vi "Setup Monthly Folders.vi"() -> ()   [LabVIEW 2024]
uses:
  TypeDefs/comic--cluster.ctl
  <vilib>/addons/_JKI.lib/Serialization/JSON/JKI JSON Serialization.lvlib
  <userlib>/_OpenG.lib/string/string.llb/openg_string.lvlib
panel:
  out "multiples":string[](array[string])
  out "status":string
  out "error out":errorcluster
  in  "comic repo":path=path "D:/Comics/Marvel"
  in  "error in":errorcluster
  in  "path":path=path "D:/data/comics"
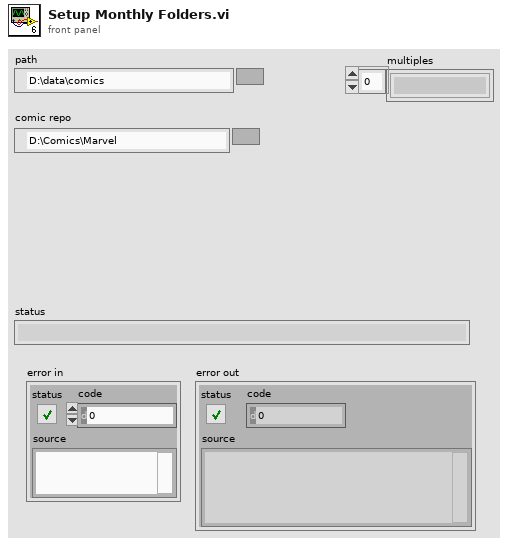
[diagram p1: front panel]
types:
  T1 = typedef "comic--cluster.ctl" = cluster{"id":i32, "digitalId":i32, "title":string, "issueNumber":i32, "variantDescription":string, "description":string, "modified":variant, "upc":string, "format":string, "pageCount":i32, "resourceURI":string, "urls":cluster{"type":string, "url":string}[], "series":cluster{"resourceURI":string, "name":string}, "dates":cluster{"type":string, "date":string}[], "prices":cluster{"price":dbl, "type":string}[], "thumbnail":cluster{"path":string, "extension":string}, "images":cluster{"path":string, "extension":string}[], "creators":cluster{"available":i32, "returned":i32, "collectionURI":string, "items":cluster{"resourceURI":string, "name":string, "role":string}[]}, "characters":cluster{"available":i32, "returned":i32, "collectionURI":string, "items":cluster{"resourceURI":string, "name":string}[]}, "stories":cluster{"available":i32, "returned":i32, "collectionURI":string, "items":cluster{"resourceURI":string, "name":string, "type":string}[]}, "events":cluster{"available":i32, "returned":i32, "collectionURI":string, "items":cluster{"resourceURI":string, "name":string}[]}}
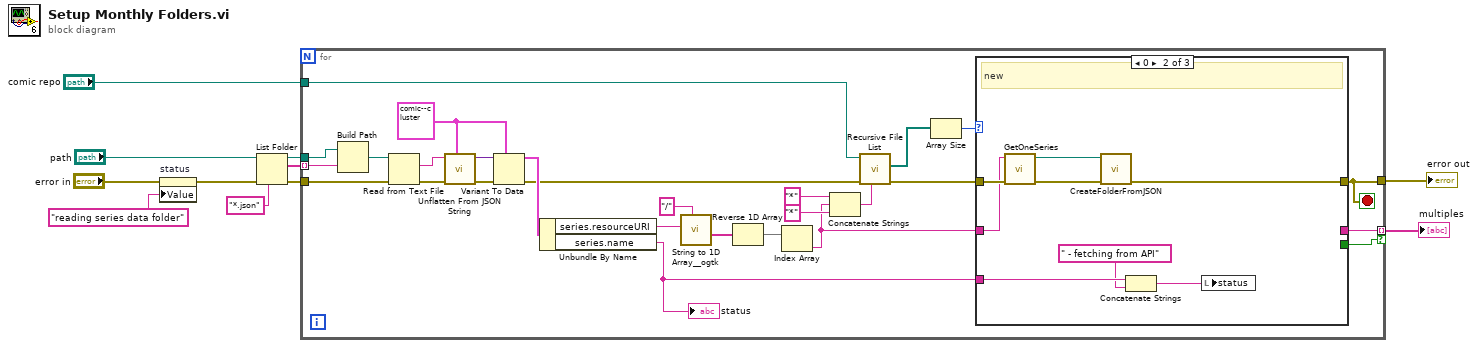
[diagram p0: block diagram]
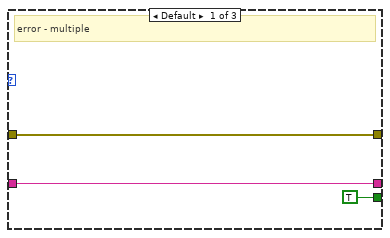
[diagram p2: hidden frame]
diagram:
  n1 = property on="status" class="Str"(error in="error in", "Value"="reading series data folder" ("status")) -> (error out=w2:errorcluster)  [unwired: 1 in, 1 out]
  n2 = List Folder(path="path", pattern="*.json", error in=w2) -> (path out=w7:path, filenames=w8:string[], error out=w9:errorcluster)  [unwired: 1 in, 1 out]
  n3 = for {
    tunnel: w9 -> [w36]
    tunnel: w8 -> [w38] mode=indexing
    tunnel: w7 -> [w37]
    tunnel: "comic repo" -> [w23]
    tunnel: [w16] -> w4
    tunnel: [w14] -> w5 mode=indexing if=w13
    stop <- w16 stop-if-true
    w30 = T1 {"id"=0, "digitalId"=0, "title"="", "issueNumber"=0, "variantDescription"="", "description"="", "modified"=variant, "upc"="", "format"="", "pageCount"=0, "resourceURI"="", "urls"=[], "series"={"resourceURI"="", "name"=""}, "dates"=[], "prices"=[], "thumbnail"={"path"="", "extension"=""}, "images"=[], "creators"={"available"=0, "returned"=0, "collectionURI"="", "items"=[]}, "characters"={"available"=0, "returned"=0, "collectionURI"="", "items"=[]}, "stories"={"available"=0, "returned"=0, "collectionURI"="", "items"=[]}, "events"={"available"=0, "returned"=0, "collectionURI"="", "items"=[]}} ("Cluster")
    n4 = Build Path(base path=w37, name or relative path=w38) -> (appended path=w35:path)
    n5 = Read from Text File(file (use dialog)=w35, error in=w36) -> (text=w33:string, error out=w34:errorcluster)  [unwired: 2 in, 2 out]
    n6 = call <vilib>:"Unflatten From JSON String.vi"("Type and Defaults"=w30, "error in (no error)"=w34, "JSON String"=w33) -> ("error out"=w32:errorcluster, "Variant"=w31:variant)  [unwired: 7 in]
    n7 = Variant To Data(error in=w32, type=w30, Variant=w31) -> (data=w29:T1, error out=w24:errorcluster)
    n8 = Unbundle By Name(w29) -> ("series.resourceURI"=w28:string, "series.name"=w12:string)
    "status" <- w12
    n9 = call <userlib>:"String to 1D Array__ogtk.vi"("delimiter (Tab)"="/", "string"=w28) -> ("Array of Strings"=w26:string[])  [unwired: 9 in]
    n10 = Reverse 1D Array(array=w26) -> (reversed array=w25:string[])
    n11 = Index Array(array=w25) -> (element=w15:string)  [unwired: 1 in]
    n12 = Concatenate Strings("*" ("string"), w15, "*" ("string")) -> (w22:string)
    n13 = call <vilib>:"Recursive File List.vi"("pattern"=w22, "error in (no error)"=w24, "Folder Path"=w23) -> ("error out"=w17:errorcluster, "All Files in Dir"=w18:path[])  [unwired: 4 in, 3 out]
    n14 = Array Size(array=w18) -> (size(s)=w19:i32)
    n15 = case shown="0" w19 {
      tunnel: w17 -> [w41 w49 w50]
      tunnel: [w41 w45 w50] -> w16
      tunnel: w15 -> [w40 w48 _]
      tunnel: [w40 _ _] -> w14
      tunnel: [TRUE _ _] -> w13
      tunnel: w12 -> [_ w44 _]
      frame Default {
        # "error - multiple"
      }
      frame 0 {
        # "new"
        n16 = call "GetOneSeries.vi"("error in (no error)"=w49, "id"=w48) -> ("error out"=w46:errorcluster, "last path"=w47:path)  [unwired: 8 in]
        n17 = call "CreateFolderFromJSON.vi"("error in"=w46, "json file path"=w47) -> ("error out"=w45:errorcluster)  [unwired: 9 in]
        n18 = Concatenate Strings(w44, " - fetching from API") -> (w42:string)
        n19 = local write "status"(w42) -> ()
      }
      frame 1 {
        # "For now, do nothing\nLater add to index.json"
        # "exists"
      }
    }
  }
  "error out" <- w4
  "multiples" <- w5
